vi "Configure Vacuum Test.vi"(8 "error in (no error)":errorcluster) -> (0 "error out":errorcluster)   [LabVIEW 2015]
panel:
  in  "Thresholds":i32(listbox)=-1
  in  "Timing":i32(listbox)=-2
  out "Cancelled?":bool
  in  "Cancel Button":bool
  in  "OK Button":bool
  out "Test Sequence":i32(listbox)=-2
  # "Configure Vacuum Test"
  # "Each step may have a functionality test and/or a leak test\n\nA functionality test is conducted by obtaining a pressure reading (PSI) and determining whether it lies between a threshold window (Func P Max and Func P Min). \n\nA leak test is conducted by obtaining the leak rate of the pressure (PSI/s) and determining whether it lies between a threshold window (Leak P Max and Leak P Min). \nLeak P Max and Leak P Min represent the threshold window for leak tests. The units for this window are in PSI/s and are"
  # "Duration refers to the run time of each step\n\nPump ON refers to the time period that the pump is ON in each step"
  # "For a threshold that does\nnot apply, please enter N/A"
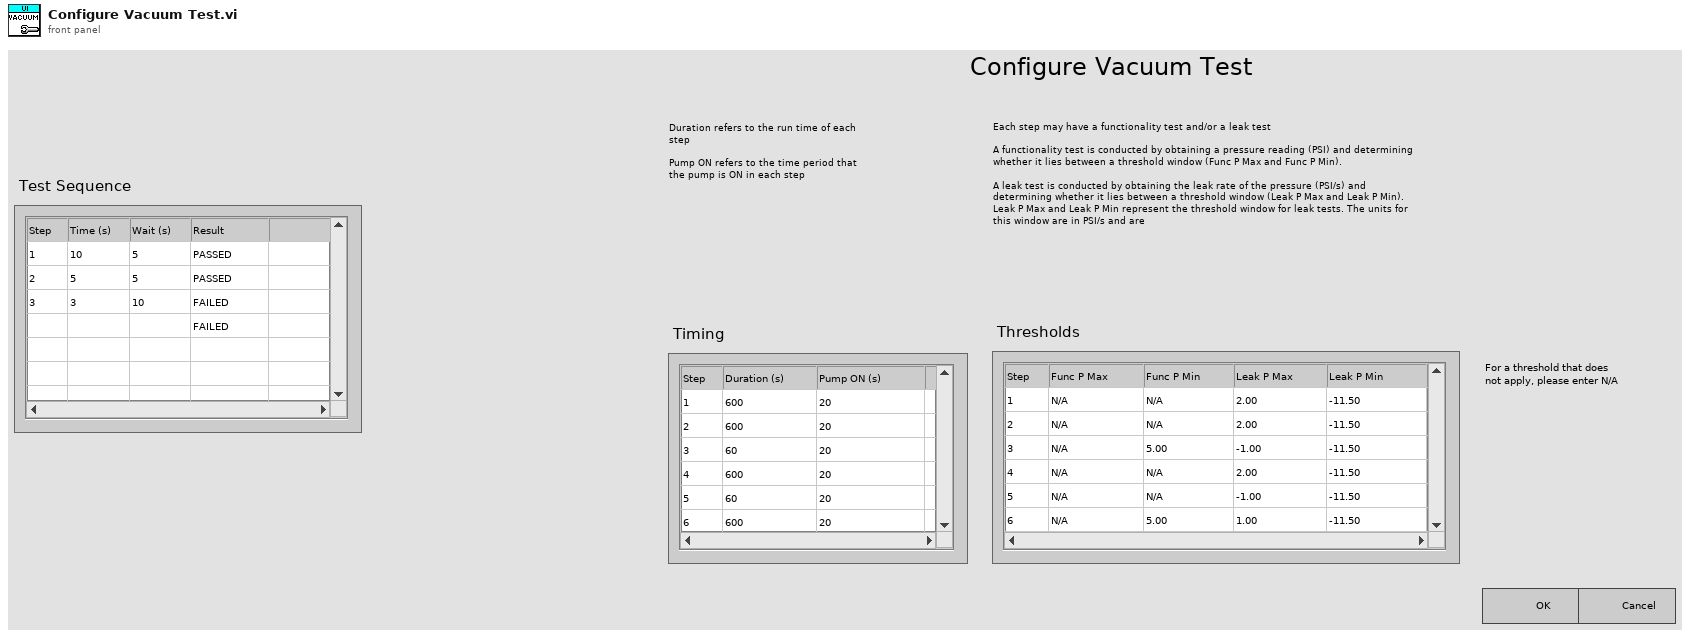
[diagram p1: front panel]
types:
  T1 = typedef "Test Information.ctl" = cluster{"Vacuum Test":T2, "Helium Test":T5, "Startup Thresholds":T7}
  T2 = typedef "Vacuum Test.ctl" = cluster{"Vacuum Timings":T3[], "Vacuum Thresholds":T4[], "Leak Reasons":string[], "Func Reasons":string[], "FuncSpecEqual":string[], "LeakSpecEqual":string[]}
  T3 = typedef "Test Timing.ctl" = cluster{"Step Wait":dbl, "Pump Wait":dbl}
  T4 = typedef "Vaccum Thresholds.ctl" = cluster{"Func Max Pressure":dbl, "Func Min Pressure":dbl, "Leak Max Pressure":dbl, "Leak Min Pressure":dbl}
  T5 = typedef "Helium Test.ctl" = cluster{"Helium Timings":T3[], "Helium Thresholds":T6[], "Failure Reasons":string[], "LeakSpecEqual":string[]}
  T6 = typedef "Helium Thresholds.ctl" = cluster{"Leak Max Pressure":dbl, "Leak Min Pressure":dbl}
  T7 = typedef "Startup Thresholds.ctl" = cluster{"MIO Max":dbl, "MIO Min":dbl, "Temp Max":dbl, "Temp Min":dbl, "Pressure Max":dbl, "Pressure Min":dbl}
  T8 = typedef "LVPoint32TypeDef.ctl" = cluster{"Horizontal":i32, "Vertical":i32}
  T9 = typedef "LVRowAndColumnTypeDef.ctl" = cluster{"Row":i32, "Column":i32}
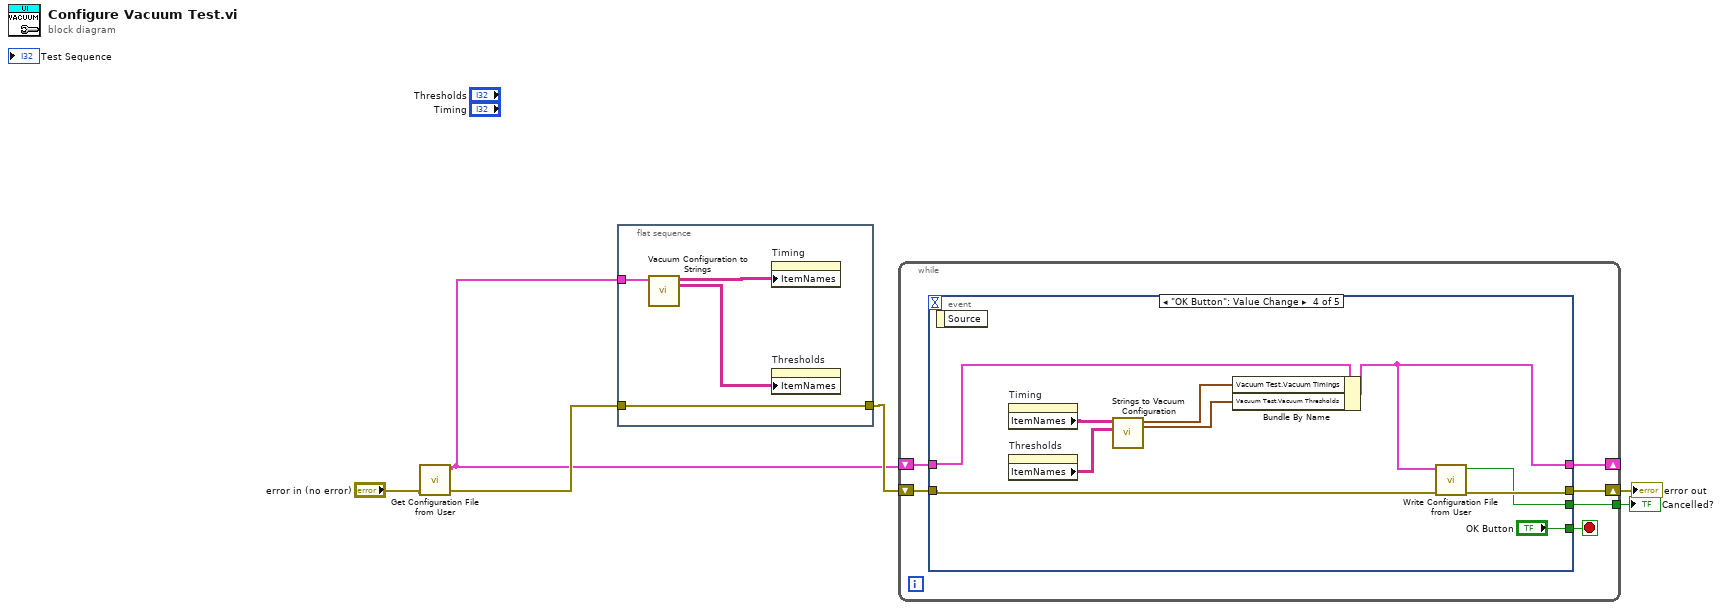
[diagram p0: block diagram]
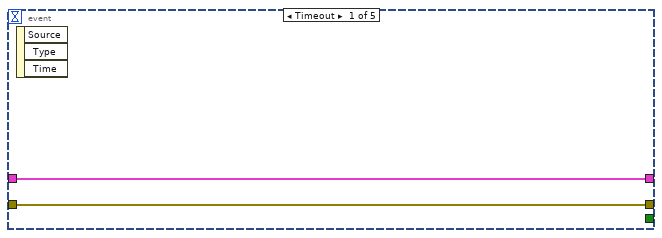
[diagram p2: hidden frame]
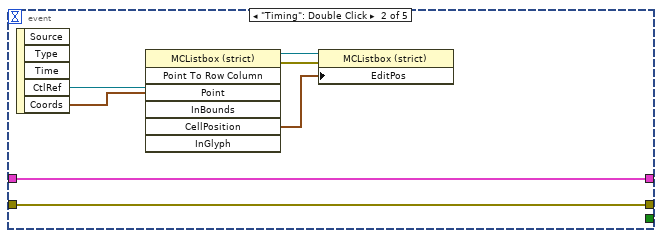
[diagram p3: hidden frame]
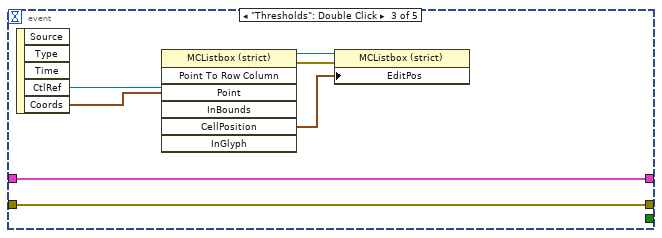
[diagram p4: hidden frame]
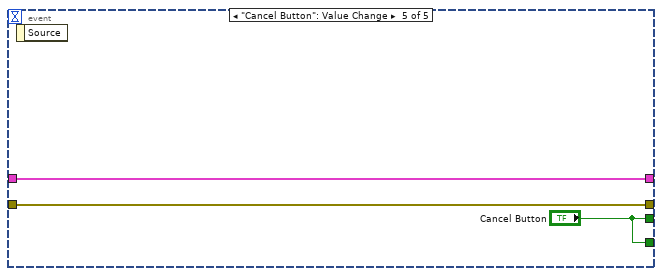
[diagram p5: hidden frame]
diagram:
  n1 = call "Get Configuration File from User.vi"("error in"="error in (no error)") -> ("error out"=w2:errorcluster, "Test Information"=w1:T1)  [unwired: 8 in, 1 out]
  n2 = flat-sequence {
    tunnel: w1 -> [w7]
    tunnel: w2 -> [w8]
    tunnel: [w8] -> w4
    frame #0 {
      n3 = call "Vacuum Configuration to Strings.vi"("Test Information"=w7) -> ("Thresholds"=w9:string[][], "Timings"=w10:string[][])  [unwired: 9 in]
      n4 = property on="Timing" class="MCListbox (strict)"("ItemNames"=w10) -> ()  [unwired: 2 in, 2 out]
      n5 = property on="Thresholds" class="MCListbox (strict)"("ItemNames"=w9) -> ()  [unwired: 2 in, 2 out]
    }
  }
  n6 = while {
    tunnel: [w16] -> w6
    shift-right: [w13] -> w5
    shift-left: w4 -> [w14]
    shift-right: [w11] -> _
    shift-left: w1 -> [w12]
    stop <- w15 stop-if-true
    n7 = event shown="[3] \"OK Button\": Value Change" {
      selector: _ -> [_ _ _ _ _]
      dyn-events: _ -> [_ _ _ _ _]
      timeout: _ -> [_ _ _ _ _]
      tunnel: [_ _ _ w34 "Cancel Button"] -> w16
      tunnel: [_ _ _ "OK Button" "Cancel Button"] -> w15
      tunnel: w14 -> [w18 w20 w27 w38 w44]
      tunnel: [w18 w20 w27 w41 w44] -> w13
      tunnel: w12 -> [w17 w19 w26 w37 w43]
      tunnel: [w17 w19 w26 w33 w43] -> w11
      event Timeout {
        n8 = event-data() -> ()  [unwired: 1 in, 3 out]
      }
      event "Timing": Double Click {
        n9 = event-data() -> ("CtlRef"=w25:refnum<vi>, "Coords"=w24:T8)  [unwired: 1 in, 3 out]
        n10 = invoke class="MCListbox (strict)" method="Point To Row Column"(reference=w25, "Point"=w24) -> (reference out=w23:refnum<vi>, error out=w22:errorcluster, "CellPosition"=w21:T9)  [unwired: 5 in, 4 out]
        n11 = property class="MCListbox (strict)"(reference=w23, error in=w22, "EditPos"=w21) -> ()  [unwired: 2 out]
      }
      event "Thresholds": Double Click {
        n12 = event-data() -> ("CtlRef"=w32:refnum<vi>, "Coords"=w31:T8)  [unwired: 1 in, 3 out]
        n13 = invoke class="MCListbox (strict)" method="Point To Row Column"(reference=w32, "Point"=w31) -> (reference out=w30:refnum<vi>, error out=w29:errorcluster, "CellPosition"=w28:T9)  [unwired: 5 in, 4 out]
        n14 = property class="MCListbox (strict)"(reference=w30, error in=w29, "EditPos"=w28) -> ()  [unwired: 2 out]
      }
      event "OK Button": Value Change {
        n15 = event-data() -> ()  [unwired: 1 in, 1 out]
        n16 = property on="Timing" class="MCListbox (strict)"() -> ("ItemNames"=w40:string[][])  [unwired: 2 in, 2 out]
        n17 = property on="Thresholds" class="MCListbox (strict)"() -> ("ItemNames"=w39:string[][])  [unwired: 2 in, 2 out]
        n18 = call "Strings to Vacuum Configuration.vi"("Thresholds"=w39, "Timings"=w40) -> ("Thresholds"=w35:T4[], "Timings"=w36:T3[])  [unwired: 8 in]
        n19 = Bundle By Name(cluster=w37, "Vacuum Test.Vacuum Timings"=w36, "Vacuum Test.Vacuum Thresholds"=w35) -> (w33:T1)
        n20 = call "Write Configuration File from User.vi"("error in"=w38, "Test Information"=w33) -> ("error out"=w41:errorcluster, "Cancelled?"=w34:bool)  [unwired: 8 in]
      }
      event "Cancel Button": Value Change {
        n21 = event-data() -> ()  [unwired: 1 in, 1 out]
      }
    }
  }
  "error out" <- w5
  "Cancelled?" <- w6
